vi "GetVideoInOptionsConfig_NET.vi"(11 ".NET Refnum in":refnum<k24>) -> (0 "error out":errorcluster, 3 "InnerText":string)   [LabVIEW 2016]
uses:
  System.Windows.Forms
panel:
  out "Table Control":string[][](table)
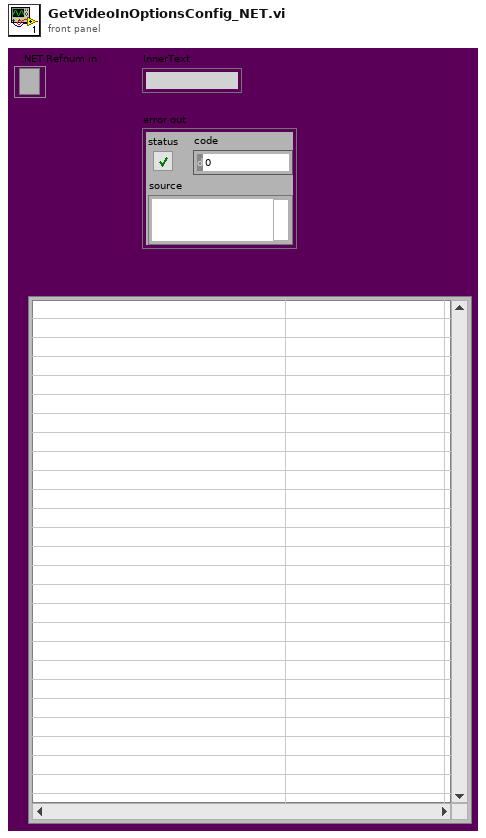
[diagram p1: front panel]
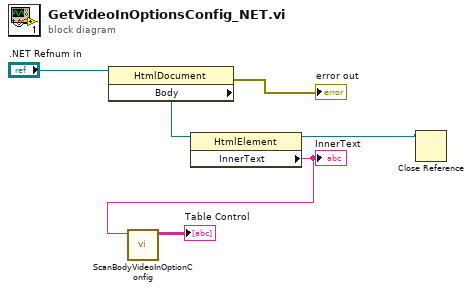
[diagram p0: block diagram]
diagram:
  n1 = property class="HtmlDocument"(reference=".NET Refnum in") -> (error out=→"error out":errorcluster, "Body"=w5:refnum<k24>)  [unwired: 1 in, 1 out]
  n2 = property class="HtmlElement"(reference=w5) -> (reference out=w1:refnum<k24>, "InnerText"=w6:string)  [unwired: 1 in, 1 out]
  "InnerText" <- w6
  n3 = call "ScanBodyVideoInOptionConfig.vi"("body"=w6) -> ("array type (2D Dbl)"=→"Table Control":string[][])  [unwired: 10 in]
  n4 = Close Reference(reference=w1) -> ()  [unwired: 1 in, 1 out]
